vi "Generate Reference File.vi"(0 "pDarkImage":u16, 1 "lpszSavePath":string, 2 "nHeight":i32, 5 "pBrightImage":u16, 7 "nBrightNum":i32, 9 "nAcqMode":i32, 11 "error in (no error)":errorcluster, 12 "nWidth":i32) -> (3 "lpszSavePath out":string, 4 "pDarkImage out":u16, 6 "pBrightImage out":u16, 8 "function return":i32, 15 "error out":errorcluster)   [LabVIEW 2017, in "imgCalibration.lvlib"]
doc: "DLLFunction int __stdcall GenerateReferenceFile(unsigned short* pDarkImage, unsigned short** pBrightImage, int nBrightNum, int nAcqMode, LPCTSTR lpszSavePath, int nWidth, int nHeight);"
uses:
  imgCalibration.lvlib
  lib/CalibrationDLL.dll
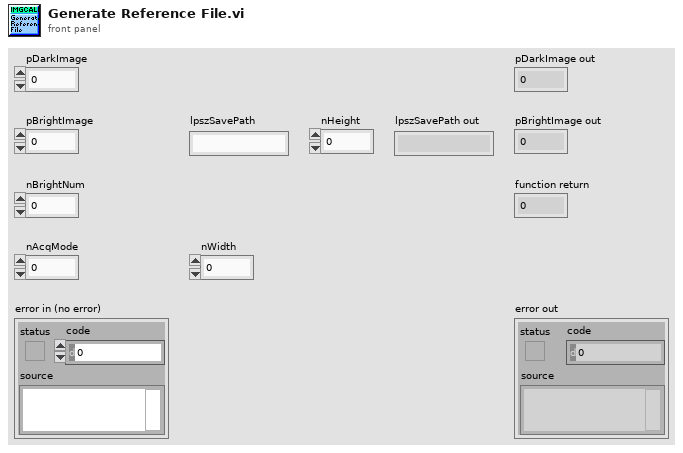
[diagram p1: front panel]
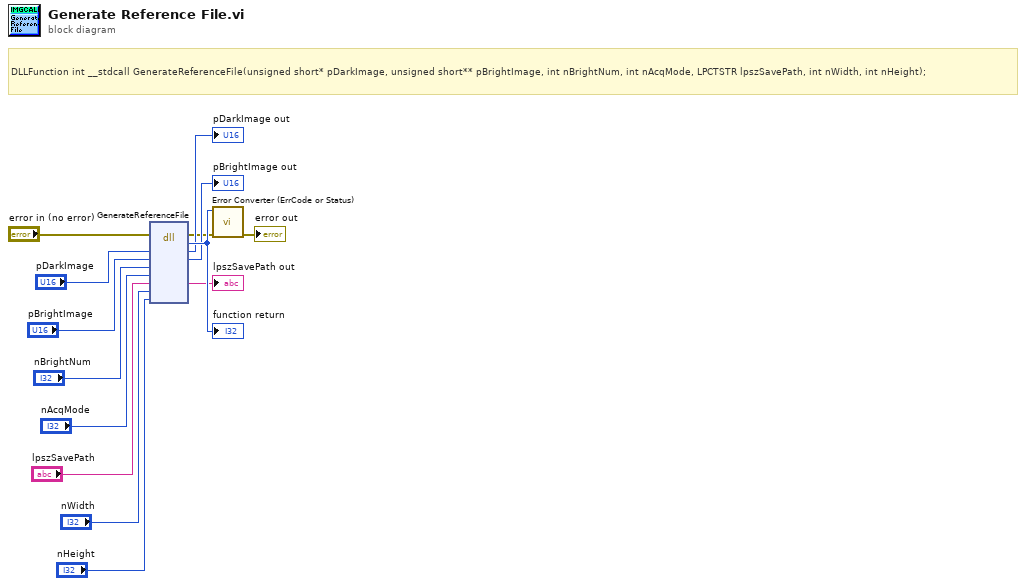
[diagram p0: block diagram]
diagram:
  # "DLLFunction int __stdcall GenerateReferenceFile(unsigned short* pDarkImage, unsigned short** pBrightImage, int nBrightNum, int nAcqMode, LPCTSTR lpszSavePath, int nWidth, int nHeight);"
  n1 = dll-call lib="F:/BonTechFlatPanelLVDriver/lib/CalibrationDLL.*" fn="GenerateReferenceFile"(error in="error in (no error)", "pDarkImage"="pDarkImage", "pBrightImage"="pBrightImage", "nBrightNum"="nBrightNum", "nAcqMode"="nAcqMode", "lpszSavePath"="lpszSavePath", "nWidth"="nWidth", "nHeight"="nHeight") -> (error out=w2:errorcluster, w14:i32, "pDarkImage"=→"pDarkImage out":u16, "pBrightImage"=→"pBrightImage out":u16, "lpszSavePath"=→"lpszSavePath out":string)  [unwired: 6 in, 1 out]
  "function return" <- w14
  n2 = call "Error Converter (ErrCode or Status).vi"("error in (no error)"=w2, "error code"=w14) -> ("error out"=→"error out":errorcluster)  [unwired: 9 in]
